vi "Configure Source.vi"(0 "VISA resource name":refnum<visa-resource-name>, 1 "Enable Continuous Output (F: Disable)":bool, 2 "Trigger Output Level (0 V)":dbl, 5 "Channel (1: Channel 1)":i32(ring)=1 items=["Channel 1"=1, "Channel 2"=2], 7 "Source Type (0: Voltage)":i32(ring) items=["Voltage"], 9 "Source Range (20 V)":dbl=20.0, 11 "error in (no error)":errorcluster, 12 "Enable Resistive Limit (F: Disable)":bool, 13 "Output Level (0 V)":dbl) -> (4 "VISA resource name out":refnum<visa-resource-name>, 15 "error out":errorcluster)   [LabVIEW 2017, in "Keysight B2980 Series.lvlib"]
doc: "Configure the output source which includes source mode, source range, output level and enables or disables the continuous output and resistive limit.\n\n<b>Note(s):</b>\nThis VI is only applicable for model B2985A and B2987A."
uses:
  Keysight B2980 Series.lvlib
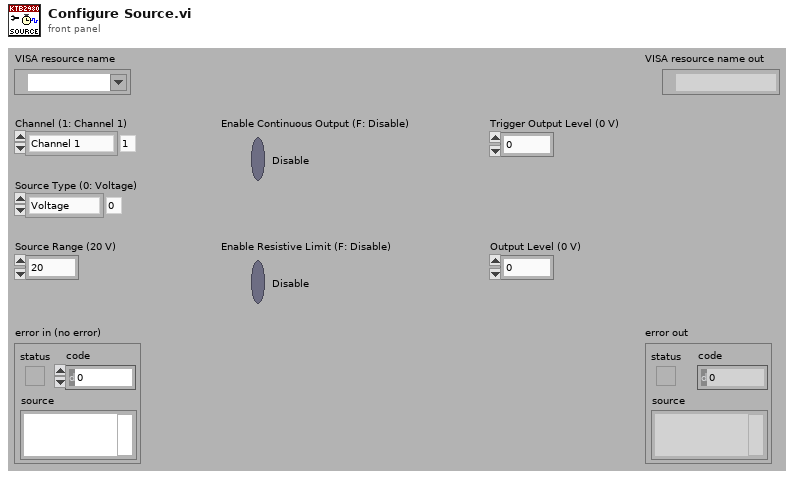
[diagram p1: front panel]
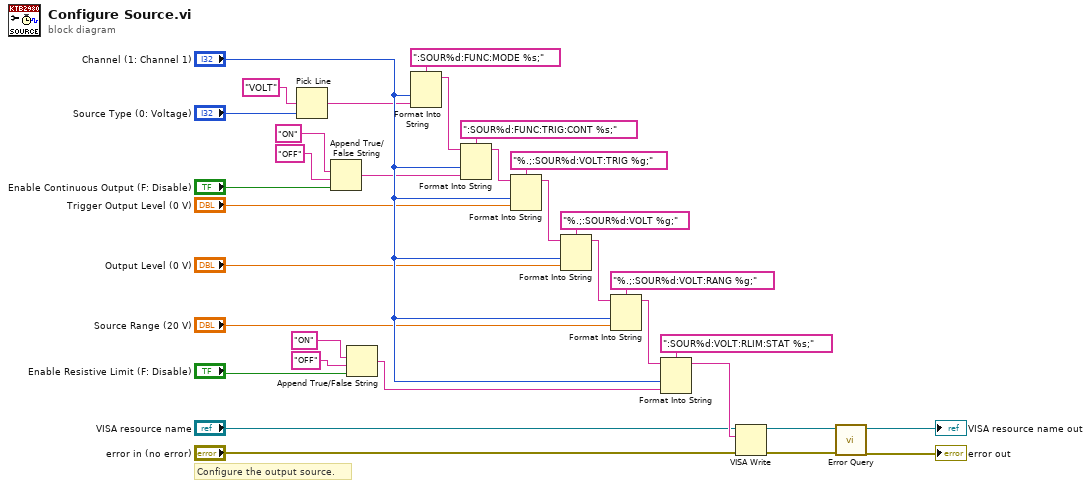
[diagram p0: block diagram]
diagram:
  # "Configure the output source."
  n1 = Pick Line(multi-line string="VOLT", line index="Source Type (0: Voltage)") -> (output string=w1:string)  [unwired: 1 out]
  n2 = Append True/False String(1:"Enable Continuous Output (F: Disable)", 2:"OFF", 3:"ON") -> (0:w26:string)  [unwired: 1 out]
  n3 = Append True/False String(1:"Enable Resistive Limit (F: Disable)", 2:"OFF", 3:"ON") -> (0:w11:string)  [unwired: 1 out]
  n4 = Format Into String(format string=":SOUR%d:FUNC:MODE %s;", "Channel (1: Channel 1)", w1) -> (resulting string=w28:string)  [unwired: 2 in, 1 out]
  n5 = Format Into String(format string=":SOUR%d:FUNC:TRIG:CONT %s;", initial string=w28, "Channel (1: Channel 1)", w26) -> (resulting string=w25:string)  [unwired: 1 in, 1 out]
  n6 = Format Into String(format string="%.;:SOUR%d:VOLT:TRIG %g;", initial string=w25, "Channel (1: Channel 1)", "Trigger Output Level (0 V)") -> (resulting string=w22:string)  [unwired: 1 in, 1 out]
  n7 = Format Into String(format string="%.;:SOUR%d:VOLT %g;", initial string=w22, "Channel (1: Channel 1)", "Output Level (0 V)") -> (resulting string=w19:string)  [unwired: 1 in, 1 out]
  n8 = Format Into String(format string="%.;:SOUR%d:VOLT:RANG %g;", initial string=w19, "Channel (1: Channel 1)", "Source Range (20 V)") -> (resulting string=w13:string)  [unwired: 1 in, 1 out]
  n9 = Format Into String(format string=":SOUR%d:VOLT:RLIM:STAT %s;", initial string=w13, "Channel (1: Channel 1)", w11) -> (resulting string=w10:string)  [unwired: 1 in, 1 out]
  n10 = VISA Write(VISA resource name="VISA resource name", write buffer=w10, error in (no error)="error in (no error)") -> (VISA resource name out=w7:refnum<visa-resource-name>, error out=w6:errorcluster)  [unwired: 1 out]
  n11 = call "Error Query.vi"("error in (no error)"=w6, "VISA resource name"=w7) -> ("error out"=→"error out":errorcluster, "VISA resource name out"=→"VISA resource name out":refnum<visa-resource-name>)  [unwired: 8 out]
